vi "get_state.vi"(8 "error in (no error)":errorcluster caption="错误输入（无错误）", 11 "LimitSwitch输入":refnum<class "LimitSwitch.lvclass">) -> (0 "error out":errorcluster caption="错误输出", 2 "state":bool, 3 "LimitSwitch输出":refnum<class "LimitSwitch.lvclass">)   [LabVIEW 2016, in "MotionControl.lvlib" / "LimitSwitch.lvclass"]
uses:
  <userlib>/MotionControl/LimitSwitch/LimitSwitch.lvclass
  <userlib>/MotionControl/LimitSwitch/LimitSwitch.lvclass/LimitSwitch.ctl
  <userlib>/UISimCanFunc_wrapper/UISimCanFunc_wrapper.lvlib
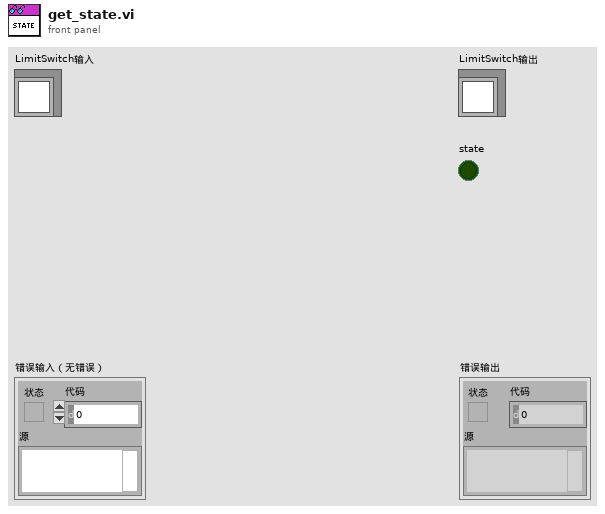
[diagram p1: front panel]
types:
  T1 = typedef "MotionControl.lvlib/LimitSwitch.lvclass/LM_ID.ctl" = i32
  T2 = typedef "UISimCanFunc_wrapper.lvlib/SFBK_INFO_OBJ.ctl" = cluster{"bSensor1":bool, "bSensor2":bool, "bSensor3":bool, "fAnaInput":sgl}
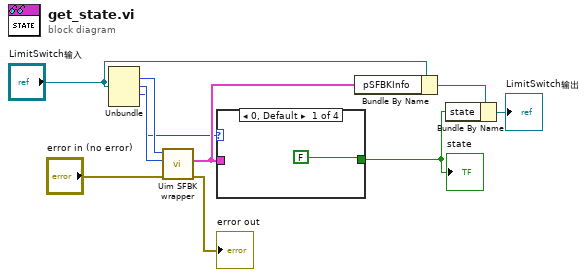
[diagram p0: block diagram]
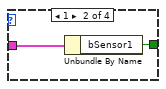
[diagram p2: hidden frame]
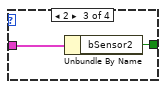
[diagram p3: hidden frame]
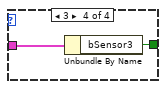
[diagram p4: hidden frame]
diagram:
  n1 = Unbundle("LimitSwitch输入") -> (w8:u32, w7:u32, w1:T1)  [unwired: 2 out]
  n2 = call <userlib>:"Uim SFBK wrapper.vi"("error in (no error)"="error in (no error)", "dwCanNodeId"=w7, "dwDevIndex"=w8) -> ("error out"=→"error out":errorcluster, "SFBK_INFO_OBJ"=w6:T2)  [unwired: 6 in, 1 out]
  n3 = case shown="0, Default" w1 {
    tunnel: w6 -> [_ w13 w15 w17]
    tunnel: [FALSE w12 w14 w16] -> w2
    frame 0, Default {
    }
    frame 1 {
      n4 = Unbundle By Name(w13) -> ("bSensor1"=w12:bool)
    }
    frame 2 {
      n5 = Unbundle By Name(w15) -> ("bSensor2"=w14:bool)
    }
    frame 3 {
      n6 = Unbundle By Name(w17) -> ("bSensor3"=w16:bool)
    }
  }
  "state" <- w2
  n7 = Bundle By Name(cluster="LimitSwitch输入", "pSFBKInfo"=w6) -> (w4:refnum<class "LimitSwitch.lvclass">)
  n8 = Bundle By Name(cluster=w4, "state"=w2) -> (→"LimitSwitch输出":refnum<class "LimitSwitch.lvclass">)
